vi "Terminal-PressureSystem-DeviceLubricateUnit-ParametersSetter.vi"(8 "error in (no error)":errorcluster caption="错误输入（无错误）", 10 "高低压供油选择":enum16{"低压供油", "高压供油"}(ring), 11 "write operation timeout (ms)":i32=5000 caption="写操作超时（5000毫秒）") -> (0 "error out":errorcluster caption="错误输出")   [LabVIEW 2014]
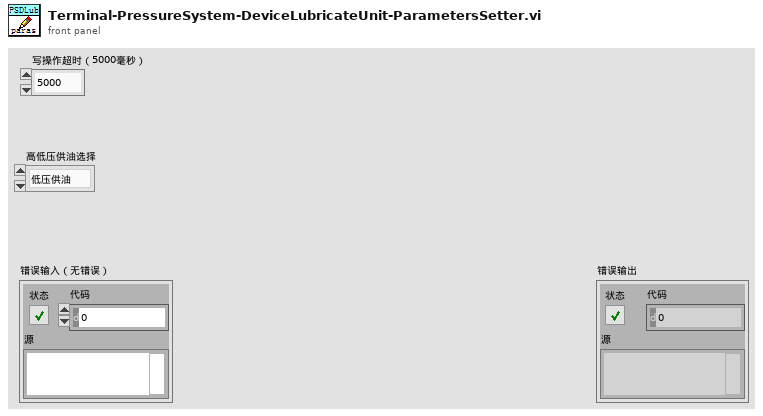
[diagram p1: front panel]
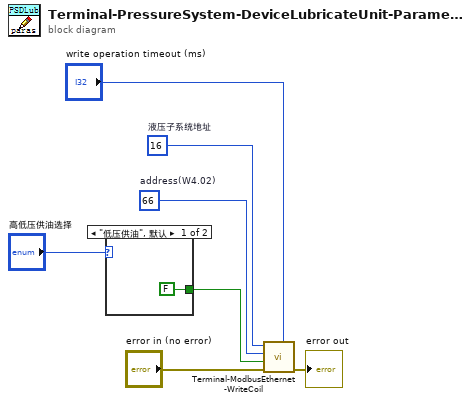
[diagram p0: block diagram]
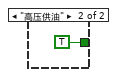
[diagram p2: hidden frame]
diagram:
  w4 = u16 66  # address(W4.02)
  w5 = u8 16  # 液压子系统地址
  n1 = case shown="\"低压供油\", 默认" "高低压供油选择" {
    tunnel: [FALSE TRUE] -> w1
    frame "低压供油", Default {
    }
    frame "高压供油" {
    }
  }
  n2 = call "Terminal-ModbusEthernet-WriteCoil.vi"("write operation timeout (ms)"="write operation timeout (ms)", "error in"="error in (no error)", "coil value"=w1, "address"=w4, "unit ID"=w5) -> ("error out"=→"error out":errorcluster)  [unwired: 6 in]
